vi "FlatToRichniswitch_grpc_SetPathRequest.vi"(5 "OutputClusterType":T1, 11 "InputCluster":T3) -> (3 "OutputCluster":T1)   [LabVIEW 2021, in "NI Switch_client.lvlib"]
uses:
  NI Switch_client.lvlib
  nidevice_grpc_Session.ctl
  niswitch_grpc_SetPathRequest.ctl
  nidevice_grpc_Session_Flat.ctl
  niswitch_grpc_SetPathRequest_Flat.ctl
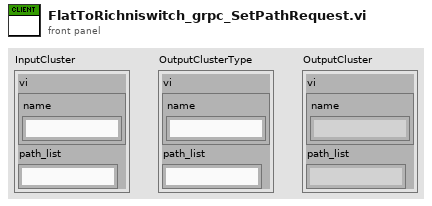
[diagram p1: front panel]
types:
  T1 = typedef "NI Switch_client.lvlib/niswitch_grpc_SetPathRequest.ctl" = cluster{"vi":T2, "path_list":string}
  T2 = typedef "NI Switch_client.lvlib/nidevice_grpc_Session.ctl" = cluster{"name":string}
  T3 = typedef "NI Switch_client.lvlib/niswitch_grpc_SetPathRequest_Flat.ctl" = cluster{"vi":T4, "path_list":string}
  T4 = typedef "NI Switch_client.lvlib/nidevice_grpc_Session_Flat.ctl" = cluster{"name":string}
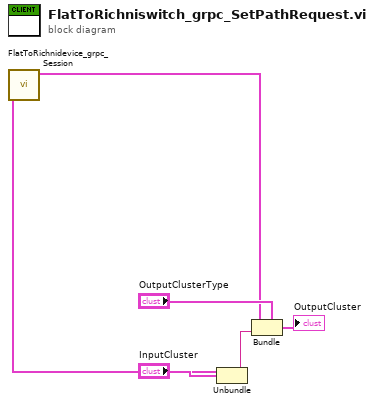
[diagram p0: block diagram]
diagram:
  n1 = Unbundle "Unbundle"("InputCluster") -> ("vi"=w3:T4, "path_list"=w1:string)
  n2 = call "FlatToRichnidevice_grpc_Session.vi"("InputCluster"=w3) -> ("OutputCluster"=w2:T2)  [unwired: 10 in]
  n3 = Bundle "Bundle"(cluster="OutputClusterType", "vi"=w2, "path_list"=w1) -> (→"OutputCluster":T1)
